vi "dt_i to 0-t_i.vi"(5 "DIO64 Debug":T1(array[cluster])) -> (0 "output cluster":cluster{bool[][], bool[][], bool[][], bool[][]}, 1 "DIOArray out 1":bool[][](array[boolean])=[[FALSE, FALSE, FALSE, FALSE, FALSE, FALSE, FALSE, FALSE, FALSE, FALSE, FALSE, FALSE, FALSE, FALSE, FALSE, FALSE], [FALSE, FALSE, FALSE, FALSE, FALSE, FALSE, FALSE, FALSE, FALSE, FALSE, FALSE, FALSE, FALSE, FALSE, FALSE, FALSE], [FALSE, FALSE, FALSE, FALSE, FALSE, FALSE, TRUE, FALSE, FALSE, FALSE, FALSE, FALSE, FALSE, FALSE, FALSE, FALSE], [FALSE, FALSE, FALSE, FALSE, FALSE, FALSE, FALSE, FALSE, FALSE, FALSE, FALSE, FALSE, FALSE, FALSE, FALSE, FALSE], [FALSE, FALSE, FALSE, FALSE, TRUE, FALSE, FALSE, FALSE, FALSE, FALSE, FALSE, FALSE, FALSE, FALSE, FALSE, FALSE], [FALSE, FALSE, FALSE, FALSE, FALSE, FALSE, FALSE, FALSE, FALSE, FALSE, FALSE, FALSE, FALSE, FALSE, FALSE, FALSE], [FALSE, FALSE, FALSE, FALSE, FALSE, TRUE, FALSE, FALSE, FALSE, FALSE, FALSE, FALSE, FALSE, FALSE, FALSE, FALSE], [FALSE, FALSE, FALSE, FALSE, FALSE, FALSE, FALSE, FALSE, FALSE, FALSE, FALSE, FALSE, FALSE, FALSE, FALSE, FALSE], [FALSE, FALSE, FALSE, FALSE, FALSE, FALSE, FALSE, FALSE, FALSE, TRUE, FALSE, FALSE, FALSE, FALSE, FALSE, FALSE], [FALSE, FALSE, FALSE, FALSE, FALSE, FALSE, FALSE, FALSE, FALSE, FALSE, TRUE, FALSE, FALSE, FALSE, FALSE, FALSE], [FALSE, FALSE, FALSE, TRUE, FALSE, FALSE, FALSE, FALSE, FALSE, FALSE, FALSE, FALSE, FALSE, FALSE, FALSE, FALSE], [FALSE, FALSE, FALSE, FALSE, FALSE, FALSE, FALSE, FALSE, FALSE, FALSE, FALSE, FALSE, FALSE, FALSE, FALSE, FALSE], [FALSE, FALSE, FALSE, FALSE, FALSE, FALSE, FALSE, TRUE, FALSE, FALSE, FALSE, FALSE, FALSE, FALSE, FALSE, FALSE], [FALSE, FALSE, FALSE, FALSE, FALSE, FALSE, FALSE, FALSE, FALSE, FALSE, FALSE, FALSE, FALSE, FALSE, FALSE, FALSE]], 2 "ti":dbl[](array[numeric]))   [LabVIEW 2012]
doc: "Creates a time array starting at 0\nadding the N time intervalls dt\nand\nAdds a Line of \"F\" to the DIO-Array\nto set all DIO-Lines to Zero at the end of the Sequence.\n\nThe size of the result array is N+1."
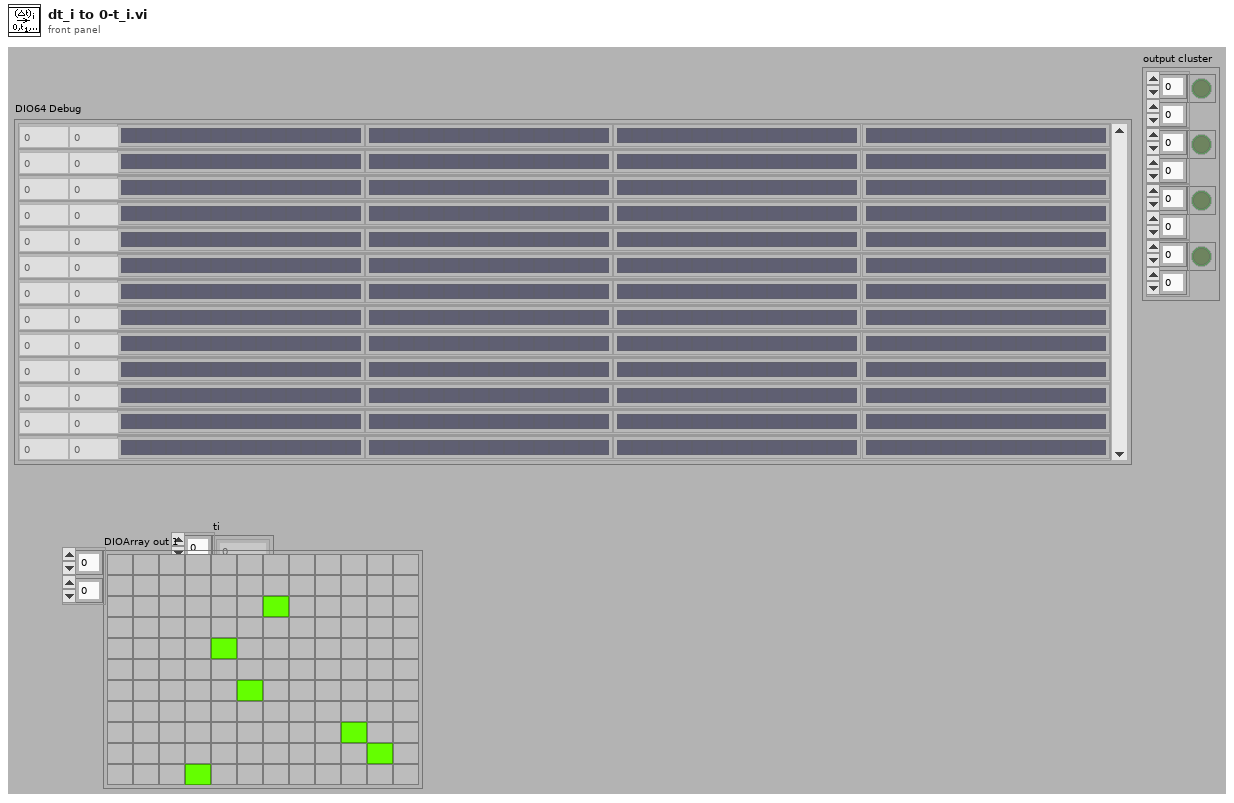
[diagram p1: front panel]
types:
  T1 = cluster{"Begin (ms)":dbl, "Duration (ms)":dbl, "DIO64 Line 1":bool[], "DIO64 Line 2":bool[], "DIO64 Line 3":bool[], "DIO64 Line 4":bool[]}[]
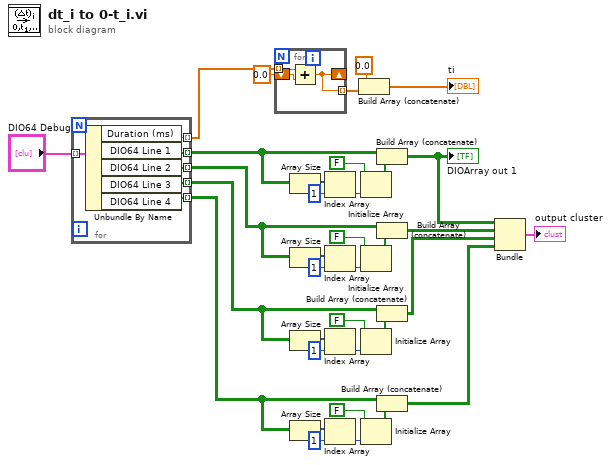
[diagram p0: block diagram]
diagram:
  n1 = for {
    tunnel: "DIO64 Debug" -> [w41] mode=indexing
    tunnel: [w40] -> w18 mode=indexing
    tunnel: [w39] -> w25 mode=indexing
    tunnel: [w38] -> w19 mode=indexing
    tunnel: [w37] -> w7 mode=indexing
    tunnel: [w36] -> w6 mode=indexing
    n2 = Unbundle By Name(w41) -> ("Duration (ms)"=w40:dbl, "DIO64 Line 1"=w39:bool[], "DIO64 Line 2"=w38:bool[], "DIO64 Line 3"=w37:bool[], "DIO64 Line 4"=w36:bool[])
  }
  n3 = for {
    tunnel: w18 -> [w44] mode=indexing
    shift-right: [w42] -> _
    shift-left: 0.0 -> [w43]
    tunnel: [w42] -> w34 mode=indexing
    n4 = Add(x=w44, y=w43) -> (x+y=w42:dbl)
  }
  n5 = Array Size(array=w25) -> (size(s)=w28:i32[])
  n6 = Array Size(array=w19) -> (size(s)=w22:i32[])
  n7 = Array Size(array=w7) -> (size(s)=w15:i32[])
  n8 = Array Size(array=w6) -> (size(s)=w10:i32[])
  n9 = Index Array(array=w28, index=1) -> (element=w30:i32)
  n10 = Index Array(array=w22, index=1) -> (element=w20:i32)
  n11 = Index Array(array=w15, index=1) -> (element=w17:i32)
  n12 = Index Array(array=w10, index=1) -> (element=w8:i32)
  n13 = Build Array (concatenate)(0.0, w34) -> (→"ti":dbl[])
  n14 = Initialize Array(FALSE, w30) -> (w29:bool[])
  n15 = Initialize Array(FALSE, w20) -> (w21:bool[])
  n16 = Initialize Array(FALSE, w17) -> (w16:bool[])
  n17 = Initialize Array(FALSE, w8) -> (w9:bool[])
  n18 = Build Array (concatenate)(w25, w29) -> (w2:bool[][])
  "DIOArray out 1" <- w2
  n19 = Build Array (concatenate)(w19, w21) -> (w3:bool[][])
  n20 = Build Array (concatenate)(w7, w16) -> (w4:bool[][])
  n21 = Build Array (concatenate)(w6, w9) -> (w5:bool[][])
  n22 = Bundle(w2, w3, w4, w5) -> (→"output cluster":cluster{bool[][], bool[][], bool[][], bool[][]})  [unwired: 1 in]
